vi "FTW-Endpoint-ConnectToListener.vi"(0 "FTW-Endpoint In":refnum<class "FTW-Endpoint-TCP.lvclass">, 5 "Address":string, 9 "Timeout":i32=1000 format="%dmsec", 11 "error in":errorcluster) -> (4 "FTW-Endpoint Out":refnum<class "FTW-Endpoint-TCP.lvclass">, 6 "Actual Address":string, 15 "error out":errorcluster)   [LabVIEW 2013, in "FTW-Endpoint-TCP.lvclass"]
uses:
  FTW-Endpoint-TCP.lvclass
  FTW-Endpoint-TCP.lvclass/FTW-Endpoint-TCP.ctl
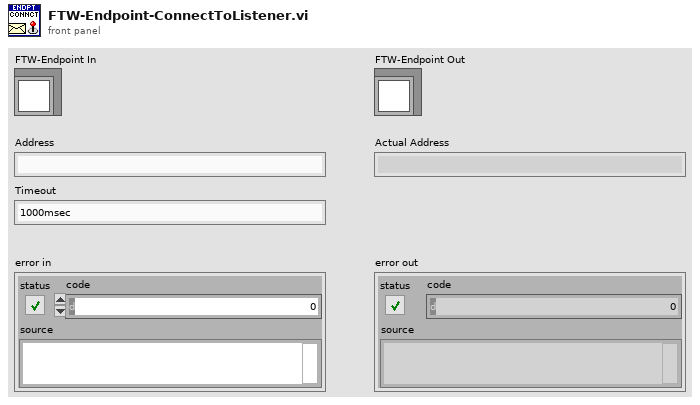
[diagram p1: front panel]
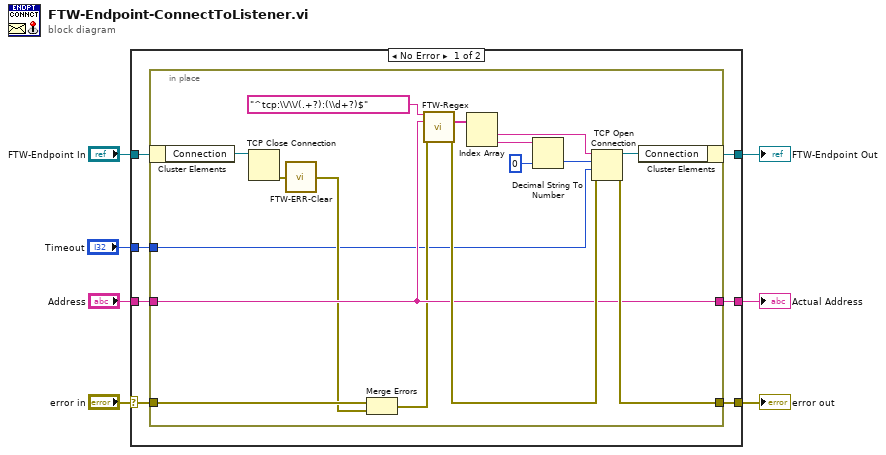
[diagram p0: block diagram]
diagram:
  n1 = case shown="No Error" "error in" {
    selector: "error in" -> [w14 w32]
    tunnel: [w13 w32] -> w7
    tunnel: [w12 w31] -> w6
    tunnel: "FTW-Endpoint In" -> [w11 w31]
    tunnel: "Address" -> [w10 _]
    tunnel: [w9 _] -> w2
    tunnel: "Timeout" -> [w8 _]
    frame No Error {
      n2 = in-place {
        in-place-border: w14 -> [w20]
        in-place-border: [w23] -> w13
        in-place-border: w10 -> [w18]
        in-place-border: [w18] -> w9
        in-place-border: w8 -> [w15]
        n3 = in-place-cluster #1(w11) -> ("Connection"=w30:refnum<k5>)
        n4 = TCP Close Connection(connection ID=w30) -> (error out=w26:errorcluster)  [unwired: 2 in, 1 out]
        n5 = call "FTW-ERR-Clear.vi"("error to snuff"=w26) -> ("no error"=w16:errorcluster)
        n6 = Merge Errors(w20, w16) -> (w17:errorcluster)
        n7 = call "FTW-Regex.vi"("Regular Expression"="^tcp:\\/\\/(.+?):(\\d+?)$" ("input string"), "Input String"=w18, "error in"=w17) -> ("Submatches"=w29:string[], "error out"=w19:errorcluster)  [unwired: 8 in, 3 out]
        n8 = Index Array(array=w29) -> (element #1=w22:string, element #2=w28:string)  [unwired: 2 in]
        n9 = Decimal String To Number(string=w28, default (0L)=u16 0 ("remote port or service name")) -> (number=w21:u16)  [unwired: 1 in, 1 out]
        n10 = TCP Open Connection(address=w22, remote port or service name=w21, timeout ms (60000)=w15, error in (no error)=w19) -> (connection ID=w24:refnum<k5>, error out=w23:errorcluster)  [unwired: 1 in]
        n11 = in-place-cluster #1("Connection"=w24) -> (w12:refnum<class "FTW-Endpoint-TCP.lvclass">)
      }
    }
    frame Error {
    }
  }
  "FTW-Endpoint Out" <- w6
  "error out" <- w7
  "Actual Address" <- w2
